vi "Read Current ProjectItem.vi"(11 "BuildManager in":refnum<class "BuildManager.lvclass">) -> (1 "Current ProjectItem":refnum<class "ProjectItem.lvclass">, 2 "Valid":bool, 3 "BuildManager out":refnum<class "BuildManager.lvclass">, 4 "In bounds":bool)   [LabVIEW 2019, in "SolutionBuilder.lvlib" / "BuildManager.lvclass"]
uses:
  BuildManager.lvclass
  ProjectItem/ProjectItem.lvclass
  BuildManager.lvclass/BuildManager.ctl
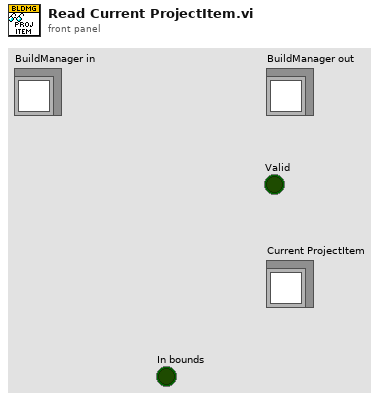
[diagram p1: front panel]
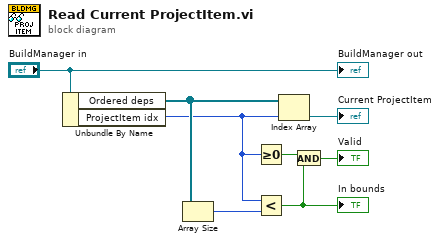
[diagram p0: block diagram]
diagram:
  n1 = Unbundle By Name("BuildManager in") -> ("Ordered deps"=w6:refnum<class "ProjectItem.lvclass">[], "ProjectItem idx"=w4:i32)
  n2 = Array Size(array=w6) -> (size(s)=w5:i32)
  n3 = Greater Or Equal To 0?(x=w4) -> (x >= 0?=w3:bool)
  n4 = Less?(x=w4, y=w5) -> (x < y?=w2:bool)
  "In bounds" <- w2
  n5 = Index Array(array=w6, index=w4) -> (element=→"Current ProjectItem":refnum<class "ProjectItem.lvclass">)
  n6 = And(x=w3, y=w2) -> (x .and. y?=→"Valid":bool)
  "BuildManager out" <- "BuildManager in"
